vi "write_angular_velocity.vi"() -> ()   [LabVIEW 2024]
uses:
  <userlib>/LabVIEW/SerialVIs/subs/portX.xctl
panel:
  in  "Linear velocities":dbl[](array[numeric])=[35.0, 0.0]
  out "2D Picture":picture
  in  "Select your port! (usbmodem101)":refnum<visa-resource-name>(xcontrol)
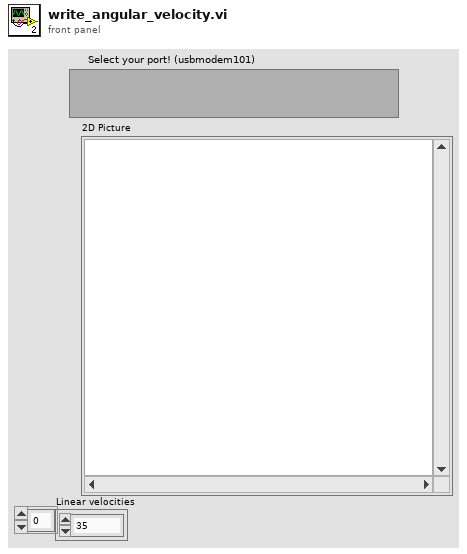
[diagram p1: front panel]
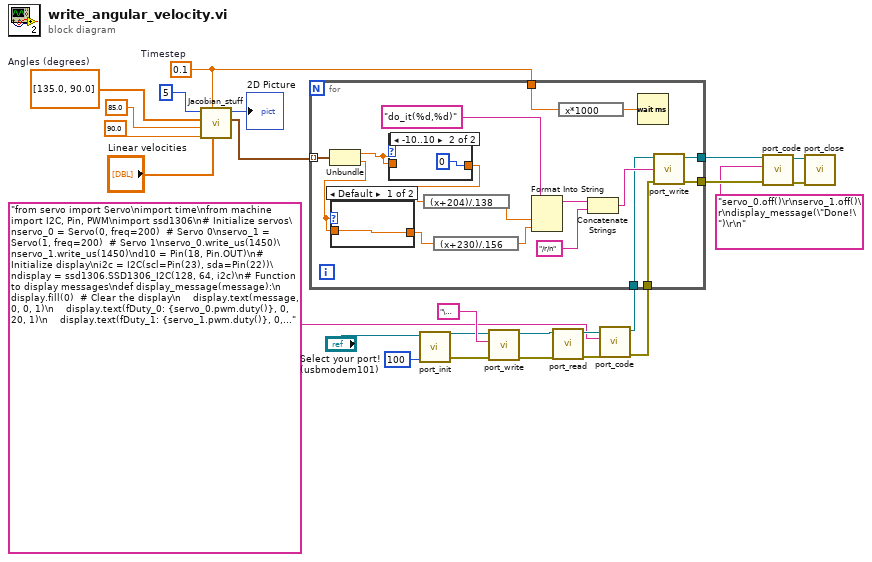
[diagram p0: block diagram]
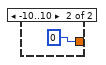
[diagram p2: hidden frame]
diagram:
  w6 = dbl[] [135.0, 90.0]  # Angles (degrees)
  w3 = 0.1  # Timestep
  n1 = call "Jacobian_stuff.vi"("Linear velocities"="Linear velocities", "Timestep"=w3, "L2"=90.0 ("L1"), "L1"=85.0, "Angles (degrees)"=w6, "Loops"=5) -> ("RPM Output\nRPM Output"=w4:cluster{dbl, dbl}[], "2D Picture"=→"2D Picture":picture)  [unwired: 4 in]
  n2 = call <userlib>:"port_init.vi"("Timeout (ms)"=u32 100, "VISA Refnum in"="Select your port! (usbmodem101)") -> ("error out"=w23:errorcluster, "VISA Refnum out"=w24:refnum<visa-resource-name>)  [unwired: 8 in]
  n3 = call <userlib>:"port_write.vi"("error in (no error)"=w23, "write buffer"="\u0003" ("CtrlC"), "VISA Refnum in"=w24) -> ("error out"=w21:errorcluster, "VISA Refnum out"=w22:refnum<visa-resource-name>)  [unwired: 7 in]
  n4 = call <userlib>:"port_read.vi"("error in (no error)"=w21, "VISA Refnum in"=w22) -> ("error out"=w18:errorcluster, "VISA Refnum out"=w17:refnum<visa-resource-name>)  [unwired: 7 in, 1 out]
  n5 = call <userlib>:"port_code.vi"("error in (no error)"=w18, "Code to run"="from servo import Servo\nimport time\nfrom machine import I2C, Pin, PWM\nimport ssd1306\n# Initialize servos\nservo_0 = Servo(0, freq=200)  # Servo 0\nservo_1 = Servo(1, freq=200)  # Servo 1\nservo_0.write_us(1450)\nservo_1.write_us(1450)\nd10 = Pin(18, Pin.OUT)\n# Initialize display\ni2c = I2C(scl=Pin(23), sda=Pin(22))\ndisplay = ssd1306.SSD1306_I2C(128, 64, i2c)\n# Function to display messages\ndef display_message(message):\n    display.fill(0)  # Clear the display\n    display.text(message, 0, 0, 1)\n    display.text(fDuty_0: {servo_0.pwm.duty()}, 0, 20, 1)\n    display.text(fDuty_1: {servo_1.pwm.duty()}, 0, 40, 1)\n    display.show()  # Update the display\ndef do_it(angle_1, angle_2):\n    servo_0.write_us(angle_1)\n    servo_1.write_us(angle_2)\n    d10.value(1)\n    time.sleep(.05)\n    d10.value(0)", "VISA Refnum in"=w17) -> ("error out"=w14:errorcluster, "VISA Refnum out"=w15:refnum<visa-resource-name>)  [unwired: 7 in]
  n6 = for {
    tunnel: w4 -> [w30] mode=indexing
    tunnel: w15 -> [w38]
    tunnel: w14 -> [w37]
    tunnel: [w36] -> w13
    tunnel: [w35] -> w12
    tunnel: w3 -> [w32]
    n7 = Unbundle(w30) -> (w29:dbl, w28:dbl)
    n8 = case shown="Default" w28 {
      tunnel: [w43 0] -> w26
      tunnel: w28 -> [w43 _]
      frame Default {
      }
      frame -10..10 {
      }
    }
    n9 = case shown="-10..10" w29 {
      tunnel: [w45 0] -> w27
      tunnel: w29 -> [w45 _]
      frame Default {
      }
      frame -10..10 {
      }
    }
    n10 = expression code="(x+204)/.138"(w27) -> (w34:dbl)
    n11 = expression code="(x+230)/.156"(w26) -> (w33:dbl)
    n12 = Format Into String(format string="do_it(%d,%d)", w34, w33) -> (resulting string=w41:string)  [unwired: 2 in, 1 out]
    n13 = expression code="x*1000"(w32) -> (w31:dbl)
    n14 = Concatenate Strings(w41, "/r/n") -> (w39:string)
    n15 = Wait (ms)(milliseconds to wait=w31) -> ()  [unwired: 1 out]
    n16 = call <userlib>:"port_write.vi"("error in (no error)"=w37, "write buffer"=w39, "VISA Refnum in"=w38) -> ("error out"=w35:errorcluster, "VISA Refnum out"=w36:refnum<visa-resource-name>)  [unwired: 7 in]
  }
  n17 = call <userlib>:"port_code.vi"("error in (no error)"=w12, "Code to run"="servo_0.off()\r\nservo_1.off()\r\ndisplay_message(\"Done!\")\r\n", "VISA Refnum in"=w13) -> ("error out"=w10:errorcluster, "VISA Refnum out"=w11:refnum<visa-resource-name>)  [unwired: 7 in]
  n18 = call <userlib>:"port_close.vi"("error in (no error)"=w10, "VISA Refnum in"=w11) -> ()  [unwired: 10 in]
